vi "Kill Pin Map Service.vi"(8 "error in":errorcluster) -> (0 "error out":errorcluster)   [LabVIEW 2020, in "MeasurementServerTests.lvlib"]
uses:
  MeasurementServerTests.lvlib
  Runtime/Measurements/Measurement Plugin Discovery V1/TypeDefs/gRPC Client Cache FGV Action.ctl
  Runtime/Measurements/Measurement Plugin Discovery V1/Measurement Plugin Discovery V1.lvlib
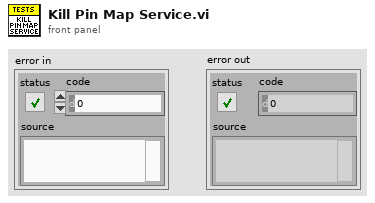
[diagram p1: front panel]
types:
  T1 = typedef "Measurement Plugin Discovery V1.lvlib/gRPC Client Cache FGV Action.ctl" = enum16{"Get Client", "Recreate Client", "Destroy Client", "Update ClusterId"}
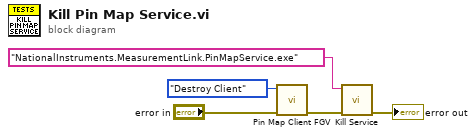
[diagram p0: block diagram]
diagram:
  n1 = call "Pin Map Client FGV.vi"("error in"="error in", "action"=gRPC_Client_Cache_FGV_Action."Destroy Client") -> ("error out"=w1:errorcluster)  [unwired: 7 in, 2 out]
  n2 = call "Kill Service.vi"("error in"=w1, "full exe name"="NationalInstruments.MeasurementLink.PinMapService.exe" ("command line")) -> ("error out"=→"error out":errorcluster)  [unwired: 9 in]
